vi "Release-notifiers.vi"(8 "error in (no error)":errorcluster, 11 "UI ref. in":refnum<data-value>) -> (0 "error out":errorcluster, 3 "UI ref.":refnum<data-value>)   [LabVIEW 2013, in "CameraVision.lvlib" / "CV-UI.lvclass"]
uses:
  CV-UI.lvclass
  CV-UI.lvclass/CV-UI.ctl
  Read Camera.vi
  Read Display-tab.vi
  Read Image refresh.vi
  Read Exit.vi
  Read Image.vi
  Read IterationTrigger.vi
  Read Mapping-characteristic.vi
  Read ScanStart.vi
  Read Settings-source.vi
  Read Acquisition.vi
  Read Acquire stop.vi
  Read Timestep.vi
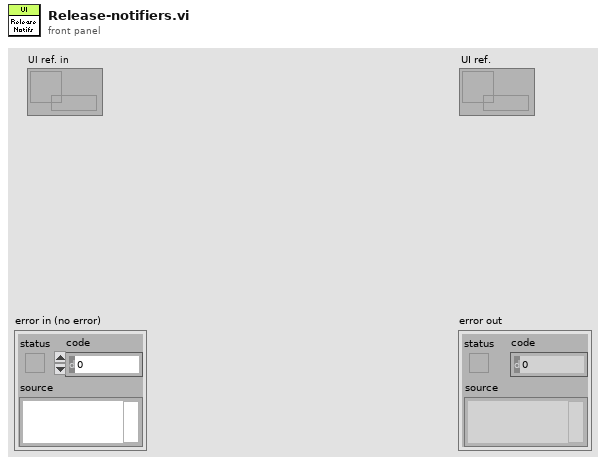
[diagram p1: front panel]
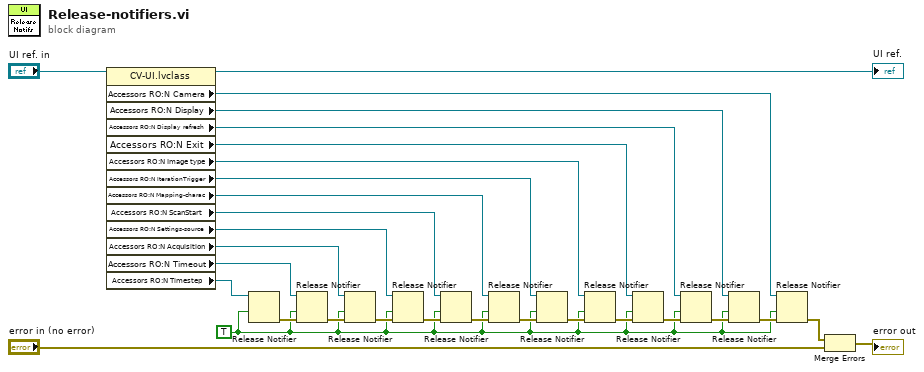
[diagram p0: block diagram]
diagram:
  w1 = TRUE
  n1 = property class="CV-UI.lvclass"(reference="UI ref. in") -> (reference out=→"UI ref.":refnum<data-value>, "Accessors RO:N Camera"=w6:refnum<notifier>, "Accessors RO:N Display"=w8:refnum<notifier>, "Accessors RO:N Display refresh"=w10:refnum<notifier>, "Accessors RO:N Exit"=w12:refnum<notifier>, "Accessors RO:N Image type"=w14:refnum<notifier>, "Accessors RO:N IterationTrigger"=w16:refnum<notifier>, "Accessors RO:N Mapping-charac"=w18:refnum<notifier>, "Accessors RO:N ScanStart"=w20:refnum<notifier>, "Accessors RO:N Settings-source"=w22:refnum<notifier>, "Accessors RO:N Acquisition"=w24:refnum<notifier>, "Accessors RO:N Timeout"=w26:refnum<notifier>, "Accessors RO:N Timestep"=w28:refnum<notifier>)  [unwired: 1 in, 1 out]
  n2 = Release Notifier(notifier=w28, force destroy? (F)=w1) -> (error out=w27:errorcluster)  [unwired: 1 in, 2 out]
  n3 = Release Notifier(notifier=w26, force destroy? (F)=w1, error in (no error)=w27) -> (error out=w25:errorcluster)  [unwired: 2 out]
  n4 = Release Notifier(notifier=w24, force destroy? (F)=w1, error in (no error)=w25) -> (error out=w23:errorcluster)  [unwired: 2 out]
  n5 = Release Notifier(notifier=w22, force destroy? (F)=w1, error in (no error)=w23) -> (error out=w21:errorcluster)  [unwired: 2 out]
  n6 = Release Notifier(notifier=w20, force destroy? (F)=w1, error in (no error)=w21) -> (error out=w19:errorcluster)  [unwired: 2 out]
  n7 = Release Notifier(notifier=w18, force destroy? (F)=w1, error in (no error)=w19) -> (error out=w17:errorcluster)  [unwired: 2 out]
  n8 = Release Notifier(notifier=w16, force destroy? (F)=w1, error in (no error)=w17) -> (error out=w15:errorcluster)  [unwired: 2 out]
  n9 = Release Notifier(notifier=w14, force destroy? (F)=w1, error in (no error)=w15) -> (error out=w13:errorcluster)  [unwired: 2 out]
  n10 = Release Notifier(notifier=w12, force destroy? (F)=w1, error in (no error)=w13) -> (error out=w11:errorcluster)  [unwired: 2 out]
  n11 = Release Notifier(notifier=w10, force destroy? (F)=w1, error in (no error)=w11) -> (error out=w9:errorcluster)  [unwired: 2 out]
  n12 = Release Notifier(notifier=w8, force destroy? (F)=w1, error in (no error)=w9) -> (error out=w7:errorcluster)  [unwired: 2 out]
  n13 = Release Notifier(notifier=w6, force destroy? (F)=w1, error in (no error)=w7) -> (error out=w3:errorcluster)  [unwired: 2 out]
  n14 = Merge Errors(w3, "error in (no error)") -> (→"error out":errorcluster)
